vi "rgb_stereo_rect.vi"(0 "Binocular Stereo Session (dup)":T3, 1 "Left image":T1, 2 "Input images":T2, 3 "error in (no error)":errorcluster, 4 "Right image":T1) -> (5 "Stereo session array (dup)":T3[](array[typedef]), 6 "Left rect image out":T1, 7 "Right rect image out":T1, 8 "error IO":errorcluster)   [LabVIEW 2019]
uses:
  <vilib>/vision/Image Controls.llb/IMAQ Image.ctl
  <vilib>/vision/Stereo.llb/IMAQ Binocular Stereo Session.ctl
  <vilib>/vision/Stereo.llb/IMAQ Binocular Reference Coordinate System.ctl
  <vilib>/vision/NI_Vision_Development_Module.lvlib
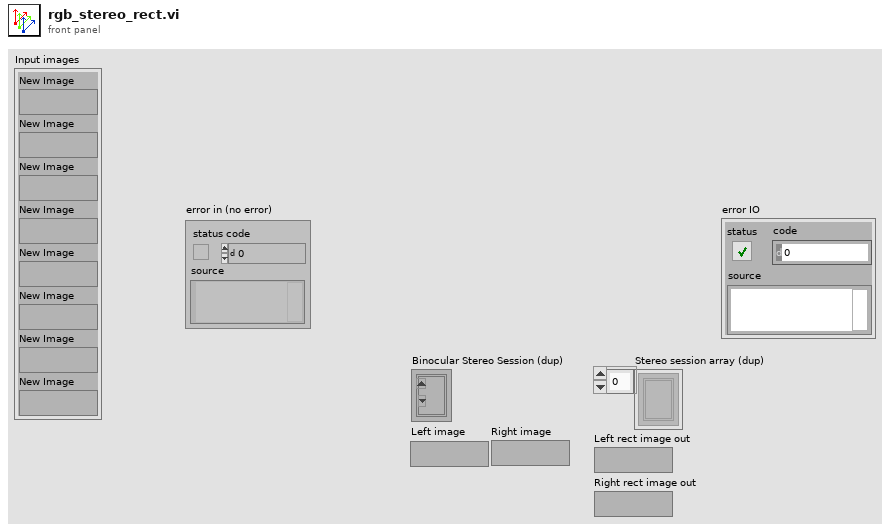
[diagram p1: front panel]
types:
  T1 = typedef "IMAQ Image.ctl" = refnum<image>
  T2 = cluster{"New Image":T1, "New Image":T1, "New Image":T1, "New Image":T1, "New Image":T1, "New Image":T1, "New Image":T1, "New Image":T1}
  T3 = typedef "IMAQ Binocular Stereo Session.ctl" = refnum<k1>
  T4 = typedef "IMAQ Binocular Reference Coordinate System.ctl" = enum32{" Left Camera", "Right Camera"}
  T5 = enum32{"Zero Order", "Bilinear", "Quadratic", "Cubic", "Bilinear Fixed"}
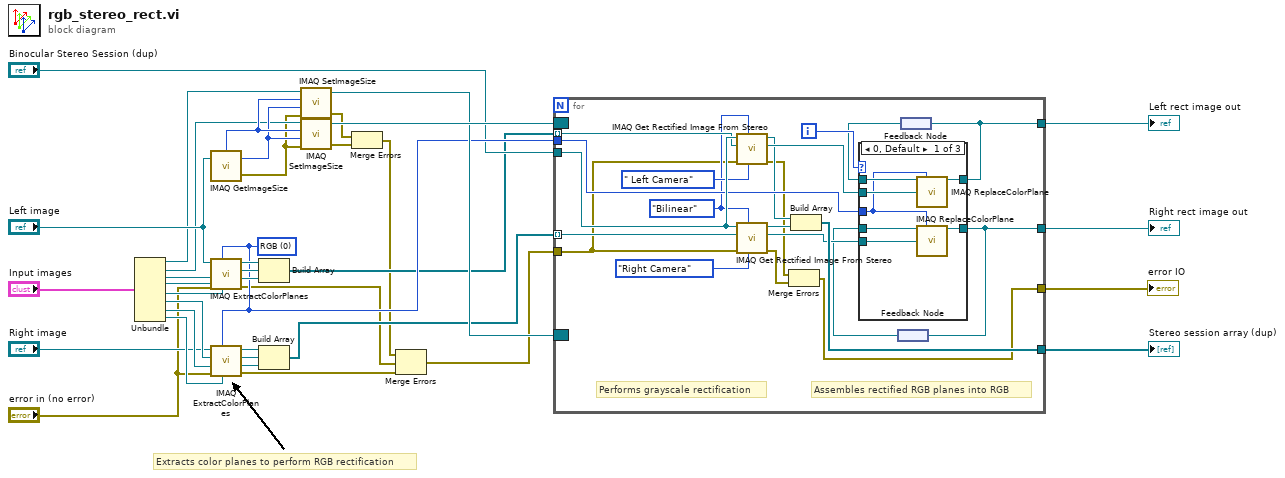
[diagram p0: block diagram]
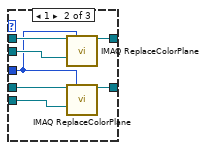
[diagram p2: hidden frame]
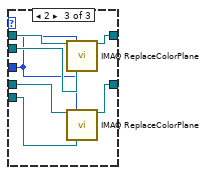
[diagram p3: hidden frame]
diagram:
  w26 = u16 0 items=["RGB", "HSL", "HSV", "HSI"] ("Color Mode")
  # "Extracts color planes to perform RGB rectification"
  n1 = Unbundle("Input images") -> ("New Image"=w12:T1, "New Image"=w11:T1, "New Image"=w10:T1, "New Image"=w9:T1, "New Image"=w8:T1, "New Image"=w5:T1, "New Image"=w6:T1, "New Image"=w7:T1)
  n2 = call "IMAQ GetImageSize"("Image"="Left image") -> ("Y Resolution"=w34:i32, "X Resolution"=w35:i32, "error out"=w2:errorcluster)  [unwired: 3 in]
  n3 = call "IMAQ ExtractColorPlanes"("Blue or Luma or Val or Inten Plane"=w8, "Color Mode"=w26, "error in (no error)"="error in (no error)", "Green or Sat Plane"=w9, "Red or Hue Plane"=w10, "Image Src"="Left image") -> ("error out"=w17:errorcluster, "Blue or Luma or Val or Inten Plane out"=w30:T1, "Green or Sat Plane out"=w31:T1, "Red or Hue Plane out"=w32:T1)  [unwired: 2 in]
  n4 = call "IMAQ ExtractColorPlanes"("Blue or Luma or Val or Inten Plane"=w7, "Color Mode"=w26, "error in (no error)"="error in (no error)", "Green or Sat Plane"=w6, "Red or Hue Plane"=w5, "Image Src"="Right image") -> ("error out"=w16:errorcluster, "Blue or Luma or Val or Inten Plane out"=w29:T1, "Green or Sat Plane out"=w28:T1, "Red or Hue Plane out"=w27:T1)  [unwired: 2 in]
  n5 = Build Array(w32, w31, w30) -> (w22:T1[])
  n6 = Build Array(w27, w28, w29) -> (w21:T1[])
  n7 = call "IMAQ SetImageSize"("error in (no error)"=w2, "Y Resolution"=w34, "X Resolution"=w35, "Image"=w12) -> ("error out"=w15:errorcluster, "Image Out"=w36:T1)  [unwired: 1 in]
  n8 = call "IMAQ SetImageSize"("error in (no error)"=w2, "Y Resolution"=w34, "X Resolution"=w35, "Image"=w11) -> ("error out"=w14:errorcluster, "Image Out"=w37:T1)  [unwired: 1 in]
  n9 = Merge Errors(w15, w14) -> (w13:errorcluster)
  n10 = Merge Errors(w13, w17, w16) -> (w20:errorcluster)
  n11 = for {
    tunnel: "Binocular Stereo Session (dup)" -> [w58]
    tunnel: [w57] -> w33
    tunnel: w22 -> [w56] mode=indexing
    tunnel: w21 -> [w55] mode=indexing
    tunnel: [w50] -> w24
    tunnel: [w49] -> w23
    tunnel: w26 -> [w47]
    border: w37 -> [_]
    border: w36 -> [_]
    tunnel: w20 -> [w41]
    tunnel: [w38] -> w19
    i -> [w54]
    w42 = T5."Bilinear" ("Interpolation Type")
    # "Assembles rectified RGB planes into RGB"
    # "Performs grayscale rectification"
    n12 = call "IMAQ Get Rectified Image From Stereo"("Reference Coordinate System"=IMAQ_Binocular_Reference_Coordinate_System." Left Camera", "Interpolation Type"=w42, "error in (no error)"=w41, "Image Src"=w56, "Binocular Stereo Session"=w58) -> ("error out"=w40:errorcluster, "Image Dst Out"=w53:T1, "Binocular Stereo Session (dup)"=w44:T3)  [unwired: 4 in]
    n13 = call "IMAQ Get Rectified Image From Stereo"("Reference Coordinate System"=IMAQ_Binocular_Reference_Coordinate_System."Right Camera", "Interpolation Type"=w42, "error in (no error)"=w41, "Image Src"=w55, "Binocular Stereo Session"=w58) -> ("error out"=w39:errorcluster, "Image Dst Out"=w52:T1, "Binocular Stereo Session (dup)"=w43:T3)  [unwired: 4 in]
    n14 = Merge Errors(w40, w39) -> (w38:errorcluster)
    n15 = Build Array(w44, w43) -> (w57:T3[])
    n16 = feedback #1() -> (w48:T1)
    n17 = feedback #2() -> (w51:T1)
    n18 = case shown="0, Default" w54 {
      tunnel: w53 -> [w61 w68 w75]
      tunnel: w52 -> [w64 w67 w74]
      tunnel: [w65 w71 w77] -> w50
      tunnel: [w63 w69 w76] -> w49
      tunnel: w51 -> [w60 w72 w79]
      tunnel: w48 -> [w62 w70 w78]
      tunnel: w47 -> [w59 w66 w73]
      frame 0, Default {
        n19 = call "IMAQ ReplaceColorPlane"("Image Src"=w60, "Color Mode"=w59, "Red or Hue Plane"=w61) -> ("Image Dst Out"=w65:T1)  [unwired: 11 in, 1 out]
        n20 = call "IMAQ ReplaceColorPlane"("Image Src"=w62, "Color Mode"=w59, "Red or Hue Plane"=w64) -> ("Image Dst Out"=w63:T1)  [unwired: 11 in, 1 out]
      }
      frame 1 {
        n21 = call "IMAQ ReplaceColorPlane"("Image Src"=w72, "Color Mode"=w66, "Green or Sat Plane"=w68) -> ("Image Dst Out"=w71:T1)  [unwired: 11 in, 1 out]
        n22 = call "IMAQ ReplaceColorPlane"("Image Src"=w70, "Color Mode"=w66, "Green or Sat Plane"=w67) -> ("Image Dst Out"=w69:T1)  [unwired: 11 in, 1 out]
      }
      frame 2 {
        n23 = call "IMAQ ReplaceColorPlane"("Image Src"=w79, "Color Mode"=w73, "Blue or Luma or Val or Inten Plane"=w75) -> ("Image Dst Out"=w77:T1)  [unwired: 11 in, 1 out]
        n24 = call "IMAQ ReplaceColorPlane"("Image Src"=w78, "Color Mode"=w73, "Blue or Luma or Val or Inten Plane"=w74) -> ("Image Dst Out"=w76:T1)  [unwired: 11 in, 1 out]
      }
    }
    n25 = feedback-in #1(w49) -> ()
    n26 = feedback-in #2(w50) -> ()
  }
  "Stereo session array (dup)" <- w33
  "Left rect image out" <- w24
  "Right rect image out" <- w23
  "error IO" <- w19
